vi "Crop Image.vi"(8 "error in (no error)":errorcluster, 10 "Crop Factor":dbl, 11 "Source Image":T1) -> (0 "error out":errorcluster, 3 "Cropped Image":T1)   [LabVIEW 2023]
uses:
  <vilib>/vision/Image Controls.llb/IMAQ Image.ctl
  Vision/Vision.lvlib
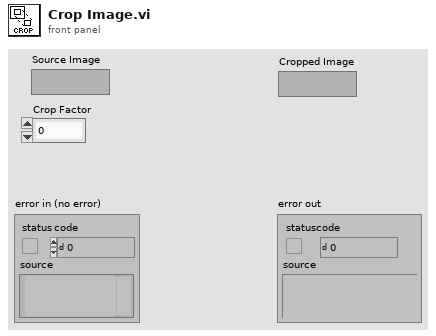
[diagram p1: front panel]
types:
  T1 = typedef "IMAQ Image.ctl" = refnum<image>
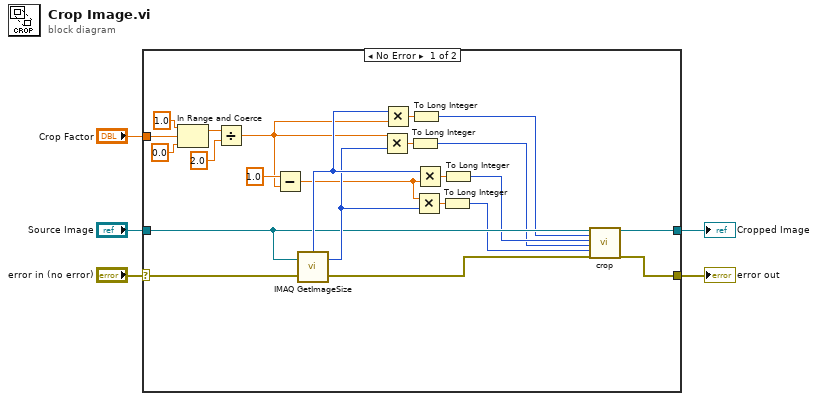
[diagram p0: block diagram]
diagram:
  n1 = case shown="No Error" "error in (no error)" {
    selector: "error in (no error)" -> [w22 w30]
    tunnel: [w12 w29] -> w1
    tunnel: [w11 w30] -> w5
    tunnel: "Source Image" -> [w13 w29]
    tunnel: "Crop Factor" -> [w21 _]
    frame No Error {
      n2 = In Range and Coerce(upper limit=1.0, x=w21, lower limit=0.0) -> (coerced(x)=w20:dbl)  [unwired: 1 out]
      n3 = Divide(x=w20, y=2.0) -> (x/y=w15:dbl)
      n4 = Subtract(x=1.0, y=w15) -> (x-y=w14:dbl)
      n5 = call "IMAQ GetImageSize"("Image"=w13, "error in (no error)"=w22) -> ("Y Resolution"=w23:i32, "X Resolution"=w24:i32, "error out"=w10:errorcluster)  [unwired: 2 in]
      n6 = Multiply(x=w15, y=w23) -> (x*y=w27:dbl)
      n7 = Multiply(x=w24, y=w15) -> (x*y=w28:dbl)
      n8 = To Long Integer(number=w27) -> (32bit integer=w7:i32)
      n9 = To Long Integer(number=w28) -> (32bit integer=w9:i32)
      n10 = Multiply(x=w14, y=w23) -> (x*y=w25:dbl)
      n11 = Multiply(x=w24, y=w14) -> (x*y=w26:dbl)
      n12 = To Long Integer(number=w25) -> (32bit integer=w6:i32)
      n13 = To Long Integer(number=w26) -> (32bit integer=w8:i32)
      n14 = call "crop.vi"("Image in"=w13, "left"=w9, "right"=w8, "top"=w7, "bottom"=w6, "error in (no error)"=w10) -> ("Image out"=w12:T1, "error out"=w11:errorcluster)  [unwired: 12 in]
    }
    frame Error {
    }
  }
  "error out" <- w5
  "Cropped Image" <- w1
